vi "Save.vi"(3 "Synapses in":refnum<class "Synapses.lvclass">) -> (0 "error out":errorcluster, 1 "Synapses out":refnum<class "Synapses.lvclass">)   [LabVIEW 2016, in "Synapses.lvclass"]
doc: "Save the synapses classe to a xml file inside the folder Results/Synapses"
uses:
  Synapses.lvclass
  Synapses.lvclass/Synapses.ctl
  <vilib>/Utility/xml.llb/Write to XML File(string).vi
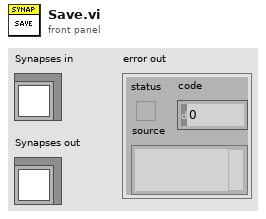
[diagram p1: front panel]
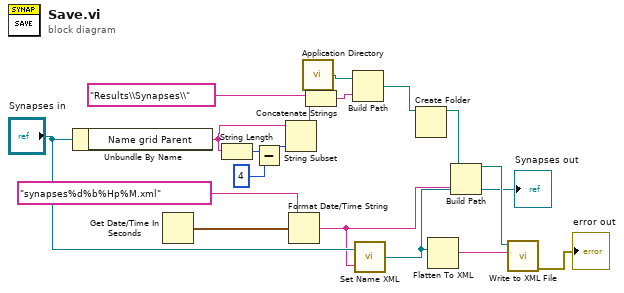
[diagram p0: block diagram]
diagram:
  n1 = Unbundle By Name("Synapses in") -> ("Name grid Parent"=w6:string)
  n2 = Get Date/Time In Seconds() -> (seconds since 1Jan1904=w17:timestamp)
  n3 = String Length(string=w6) -> (length=w7:i32)
  n4 = Subtract(x=w7, y=4) -> (x-y=w5:i32)
  n5 = String Subset(string=w6, length (rest)=w5) -> (substring=w8:string)  [unwired: 1 in]
  n6 = Format Date/Time String(time format string (%c)="synapses%d%b%Hp%M.xml", seconds (now)=w17) -> (date/time string=w2:string)  [unwired: 1 in]
  n7 = call <vilib>:"Application Directory.vi"() -> ("Application Directory"=w18:path)
  n8 = Concatenate Strings("Results\\Synapses\\" ("name or relative path"), w8) -> (w11:string)
  n9 = Build Path(base path=w18, name or relative path=w11) -> (appended path=w10:path)
  n10 = call-dynamic "Set Name XML.vi"("Name XML File"=w2, "Synapses in"="Synapses in") -> ("Synapses out"=w1:refnum<class "Synapses.lvclass">)
  "Synapses out" <- w1
  n11 = Create Folder(path (use dialog)=w10) -> (created path=w9:path)  [unwired: 2 in, 2 out]
  n12 = Flatten To XML(anything=w1) -> (xml string=w14:string)
  n13 = Build Path(base path=w9, name or relative path=w2) -> (appended path=w13:path)
  n14 = call-poly <vilib>:"Write to XML File.vi"("XML Input"=w14, "XML File Path"=w13) -> ("error out"=→"error out":errorcluster)  [unwired: 7 in, 2 out]
